vi "K Init.vi"(8 "error in (no error)":errorcluster, 9 "BaudRate":i32, 10 "Channel":u8, 11 "DevHandle":i32) -> (0 "error out":errorcluster, 3 "function return":i32)   [LabVIEW 2010, in "usb2k.lvlib"]
doc: "int WINAPI K_Init(int DevHandle, unsigned char Channel,int BaudRate);"
uses:
  usb2k.lvlib
  examples/Labview/PublicFiles/USB2XXX.dll
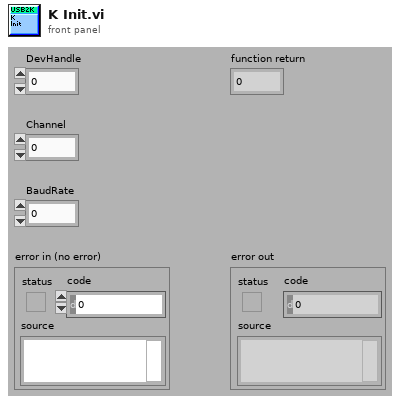
[diagram p1: front panel]
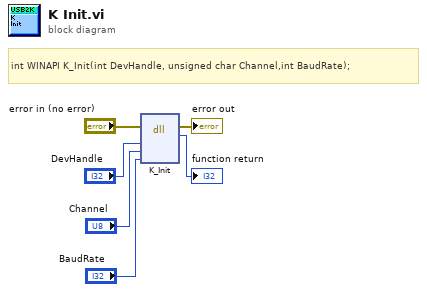
[diagram p0: block diagram]
diagram:
  # "int WINAPI K_Init(int DevHandle, unsigned char Channel,int BaudRate);"
  n1 = dll-call lib="E:/OtherWork/STM32/USB2XXX_Example/examples/Labview/PublicFiles/USB2XXX.*" fn="K_Init"(error in="error in (no error)", "DevHandle"="DevHandle", "Channel"="Channel", "BaudRate"="BaudRate") -> (error out=→"error out":errorcluster, →"function return":i32)  [unwired: 5 in, 1 out]
